vi "Get Array Values as JSON.vi"(8 "error in (no error)":errorcluster, 11 "JSON Value in":refnum<class "JSON Value.lvclass">) -> (0 "error out":errorcluster, 1 "single type?":bool, 2 "types":T1[](array[typedef]), 3 "values":refnum<class "JSON Value.lvclass">[](array[class]))   [LabVIEW 2016, in "JSON Value.lvclass"]
doc: "Returns the element type of each element in a JSON Array. If all elements are of the same type, single type is true."
uses:
  JSON Value.lvclass
  JSON Types.ctl
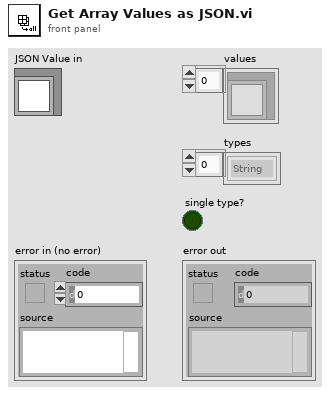
[diagram p1: front panel]
types:
  T1 = typedef "JSON Value.lvclass/JSON Types.ctl" = enum16{"String", "Numeric", "Boolean", "NULL", "Object", "Array"}
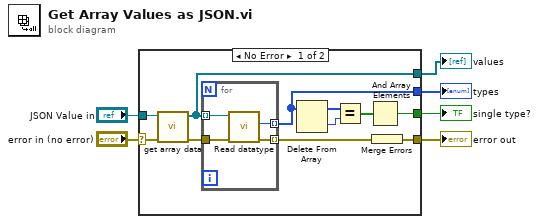
[diagram p0: block diagram]
diagram:
  n1 = case shown="No Error" "error in (no error)" {
    selector: "error in (no error)" -> [w10 w22]
    tunnel: [w7 w22] -> w5
    tunnel: "JSON Value in" -> [w17 _]
    tunnel: [w16 _] -> w3
    tunnel: [w12 _] -> w2
    tunnel: [w11 _] -> w1
    frame No Error {
      n2 = call "get array data.vi"("error in (no error)"=w10, "JSON Value in"=w17) -> ("error out"=w9:errorcluster, "JSON Array out"=w16:refnum<class "JSON Value.lvclass">[])  [unwired: 8 in]
      n3 = for {
        tunnel: w16 -> [w21] mode=indexing
        tunnel: [w20] -> w11 mode=indexing
        tunnel: w9 -> [w19]
        tunnel: [w18] -> w8 mode=indexing
        n4 = call "Read datatype.vi"("error in (no error)"=w19, "JSON Datatype in"=w21) -> ("error out"=w18:errorcluster, "datatype"=w20:T1)  [unwired: 7 in, 1 out]
      }
      n5 = Delete From Array(array=w11) -> (deleted portion=w14:T1, array with subset deleted=w15:T1[])  [unwired: 2 in]
      n6 = Equal?(x=w15, y=w14) -> (x = y?=w13:bool[])
      n7 = And Array Elements(Boolean array=w13) -> (logical AND=w12:bool)
      n8 = Merge Errors(w8) -> (w7:errorcluster)
    }
    frame Error {
    }
  }
  "error out" <- w5
  "types" <- w1
  "single type?" <- w2
  "values" <- w3
